vi "DescriptorElementsToVariantCluster.vi"(8 "Cluster Name":string, 9 "Descriptors":T1[](array[typedef])) -> (2 "Variant Cluster":variant)   [LabVIEW 2020, in "OpenDescriptor.lvlib"]
uses:
  OpenDescriptor.lvlib
  OpenDescriptor -- cluster.ctl
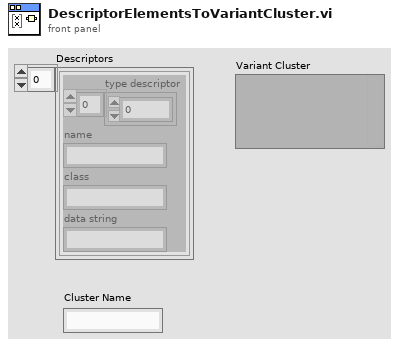
[diagram p1: front panel]
types:
  T1 = typedef "OpenDescriptor.lvlib/OpenDescriptor -- cluster.ctl" = cluster{"type descriptor":i16[], "name":string, "class":string, "data string":string}
  T2 = typedef "Type Descriptor I16 Array.ctl" = T3[]
  T3 = typedef "Type Descriptor I16.ctl" = i16
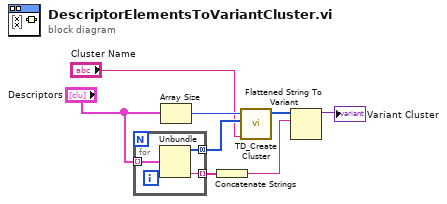
[diagram p0: block diagram]
diagram:
  n1 = for {
    tunnel: "Descriptors" -> [w11] mode=indexing
    tunnel: [w10] -> w7 mode=concatenating
    tunnel: [w9] -> w5 mode=indexing
    n2 = Unbundle(w11) -> ("type descriptor"=w10:i16[], "data string"=w9:string)  [unwired: 2 out]
  }
  n3 = Array Size(array="Descriptors") -> (size(s)=w6:i32)
  n4 = Concatenate Strings(w5) -> (w4:string)
  n5 = call <vilib>:"TD_Create Cluster.vi"("Name"="Cluster Name", "Concatenated Elts"=w7, "N Elts"=w6) -> ("ClusterTD"=w8:T2)  [unwired: 8 in]
  n6 = Flattened String To Variant(6:w4, 7:w8) -> (3:→"Variant Cluster":variant)  [unwired: 1 in, 1 out]
